vi "subReplaceSymbolValue.vi"(8 "error in (no error)":errorcluster, 9 "Value":string, 10 "Symbol":string, 11 "Project Path":path) -> (0 "error out":errorcluster, 1 "Output Message":string, 2 "Exit Code":i32)   [LabVIEW 2014, in "lvcommonbuild.lvlib"]
uses:
  lvcommonbuild.lvlib
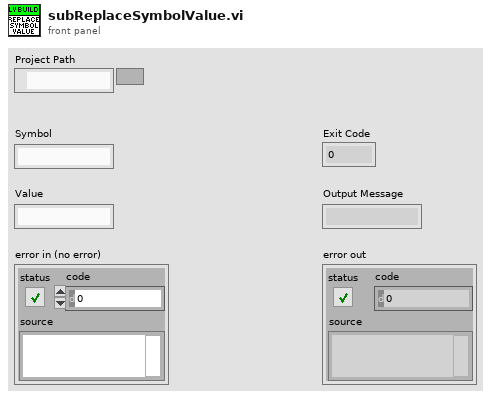
[diagram p1: front panel]
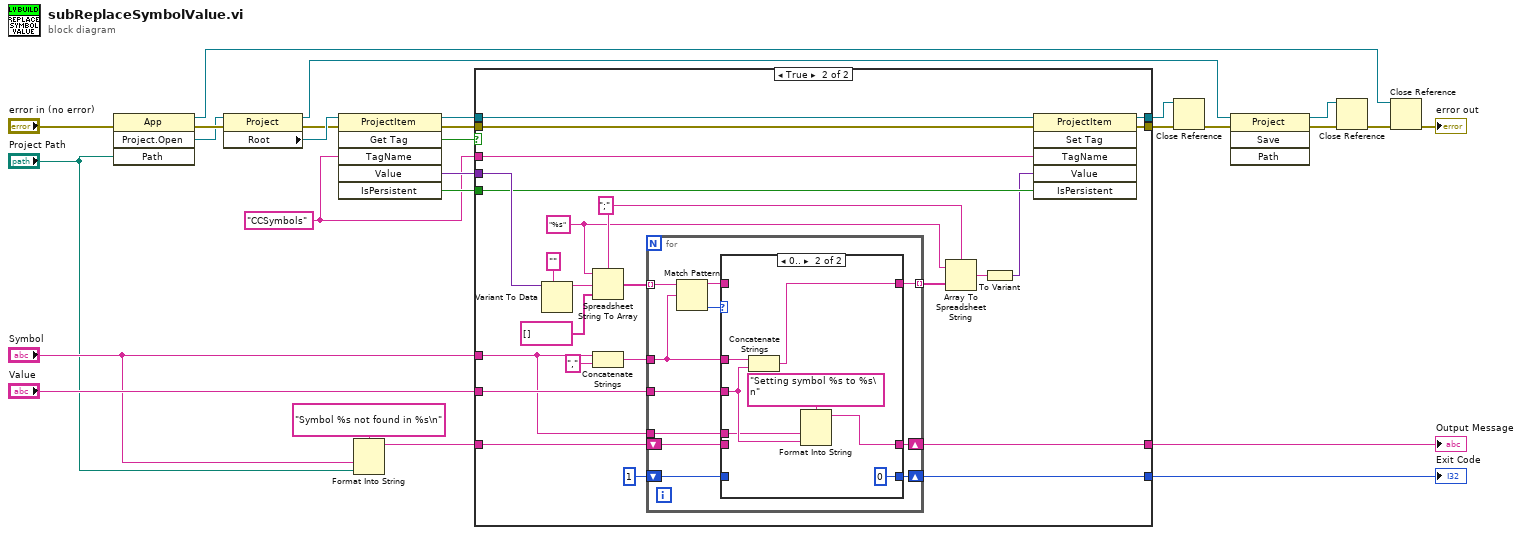
[diagram p0: block diagram]
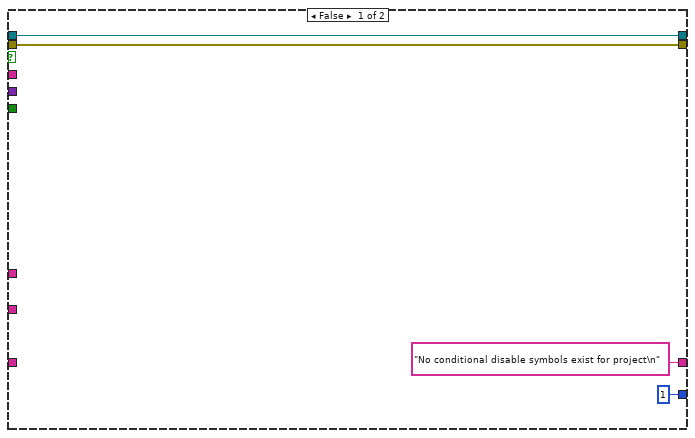
[diagram p2: hidden frame]
diagram:
  w21 = "CCSymbols" ("Tag Name")
  n1 = invoke class="App" method="Project.Open"(error in="error in (no error)", "Path"="Project Path") -> (reference out=w7:refnum<vi>, error out=w14:errorcluster, "Project:Open"=w13:refnum<vi>)  [unwired: 2 in, 1 out]
  n2 = property class="Project"(reference=w13, error in=w14) -> (reference out=w9:refnum<vi>, error out=w15:errorcluster, "Root"=w16:refnum<vi>)
  n3 = invoke class="ProjectItem" method="Get Tag"(reference=w16, error in=w15, "TagName"=w21) -> (reference out=w23:refnum<vi>, error out=w24:errorcluster, "GetTag"=w25:bool, "Value"=w26:variant, "IsPersistent"=w22:bool)  [unwired: 3 in, 1 out]
  n4 = Format Into String(format string="Symbol %s not found in %s\n" ("Tag Name"), "Symbol", "Project Path") -> (resulting string=w3:string)  [unwired: 2 in, 1 out]
  n5 = case shown="True" w25 {
    tunnel: w26 -> [_ w55]
    tunnel: "Symbol" -> [_ w35]
    tunnel: "Value" -> [_ w48]
    tunnel: w24 -> [w31 w43]
    tunnel: w23 -> [w30 w42]
    tunnel: [w31 w41] -> w11
    tunnel: [w30 w40] -> w10
    tunnel: w22 -> [_ w39]
    tunnel: w21 -> [_ w37]
    tunnel: w3 -> [_ w36]
    tunnel: ["No conditional disable symbols exist for project\n" w34] -> w2
    tunnel: [1 ("Exit Code") w33] -> w1
    frame False {
    }
    frame True {
      w45 = "%s" ("format string")
      w46 = ";" ("delimiter (Tab)")
      n6 = Variant To Data(type="", Variant=w55) -> (data=w53:string)  [unwired: 1 in, 1 out]
      n7 = Spreadsheet String To Array(delimiter (Tab)=w46, format string=w45, spreadsheet string=w53, array type (2D Dbl)=string[] []) -> (array=w51:string[])
      n8 = Concatenate Strings(w35, "," ("string")) -> (w49:string)
      n9 = for {
        tunnel: w51 -> [w65] mode=indexing
        tunnel: w49 -> [w61]
        tunnel: w48 -> [w62]
        tunnel: [w64] -> w47 mode=indexing
        shift-right: [w59] -> w34
        shift-left: w36 -> [w60]
        tunnel: w35 -> [w58]
        shift-right: [w56] -> w33
        shift-left: 1 ("Exit Code") -> [w57]
        n10 = Match Pattern(string=w65, regular expression=w61) -> (before substring=w63:string, offset past match=w66:i32)  [unwired: 1 in, 2 out]
        n11 = case shown="0.." w66 {
          tunnel: w63 -> [w69 _]
          tunnel: [w69 w75] -> w64
          tunnel: w62 -> [_ w72]
          tunnel: w61 -> [_ w76]
          tunnel: w60 -> [w68 _]
          tunnel: [w68 w73] -> w59
          tunnel: w58 -> [_ w71]
          tunnel: w57 -> [w67 _]
          tunnel: [w67 0 ("Exit Code")] -> w56
          frame Default {
          }
          frame 0.. {
            n12 = Concatenate Strings(w76, w72) -> (w75:string)
            n13 = Format Into String(format string="Setting symbol %s to %s\n", w71, w72) -> (resulting string=w73:string)  [unwired: 2 in, 1 out]
          }
        }
      }
      n14 = Array To Spreadsheet String(delimiter (Tab)=w46, array=w47, 3:w45) -> (spreadsheet string=w44:string)
      n15 = To Variant(anything=w44) -> (Variant=w38:variant)
      n16 = invoke class="ProjectItem" method="Set Tag"(reference=w42, error in=w43, "TagName"=w37, "Value"=w38, "IsPersistent"=w39) -> (reference out=w40:refnum<vi>, error out=w41:errorcluster)  [unwired: 1 in, 4 out]
    }
  }
  "Output Message" <- w2
  "Exit Code" <- w1
  n17 = Close Reference(reference=w10, error in (no error)=w11) -> (error out=w20:errorcluster)
  n18 = invoke class="Project" method="Save"(reference=w9, error in=w20) -> (reference out=w18:refnum<vi>, error out=w19:errorcluster)  [unwired: 2 in, 2 out]
  n19 = Close Reference(reference=w18, error in (no error)=w19) -> (error out=w17:errorcluster)
  n20 = Close Reference(reference=w7, error in (no error)=w17) -> (error out=→"error out":errorcluster)
